vi "TagRead.vi"(7 "LabVIEW Web Service Request":refnum<class "Web Request.lvclass">, 10 "type":string, 11 "tagName":string) -> ()   [LabVIEW 2013]
doc: "TagRead returns the value of the tag specified. Specifying the type isn't required, but results in slightly faster performance."
uses:
  <vilib>/wsapi/Web Request.lvclass
  <vilib>/NI/Tag Bus/tag/Data Type.ctl
  <vilib>/NI/Tag Bus/table/data table.ctl
  <vilib>/NI/TagWebClient/API/JSON Formats/read tag value.ctl
  <vilib>/NI/TagWebClient/API/tagweb client API.lvlib
  <vilib>/NI/Tag Bus/tag/tag descriptor.lvclass
  <vilib>/NI/Tag Bus/table/data table.lvlib
  <vilib>/NI/Tag Bus/dictionary/data dictionary.lvclass
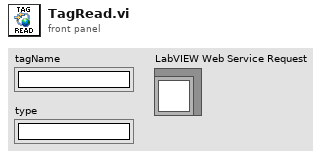
[diagram p1: front panel]
types:
  T1 = typedef "tag bus.lvlib/tag descriptor.lvclass/Data Type.ctl" = enum16{"Double", "Single", "I64", "I32", "I16", "I8", "U64", "U32", "U16", "U8", "Boolean", "String", "Array of Double", "Array of Single", "Array of I64", "Array of I32", "Array of I16", "Array of I8", "Array of U64", "Array of U32", "Array of U16", "Array of U8", "Array of Boolean", "Array of String"}
  T2 = typedef "tag bus.lvlib/data table.lvlib/data table.ctl" = cluster{"Double":dbl[], "Single":sgl[], "I64":i64[], "I32":i32[], "I16":i16[], "I8":i8[], "U64":u64[], "U32":u32[], "U16":u16[], "U8":u8[], "Boolean":bool[], "String":string[], "Array of Double":cluster{"DBL Array":dbl[]}[], "Array of Single":cluster{"SGL Array":sgl[]}[], "Array of I64":cluster{"I64 Array":i64[]}[], "Array of I32":cluster{"I32 Array":i32[]}[], "Array of I16":cluster{"I16 Array":i16[]}[], "Array of I8":cluster{"I8 Array":i8[]}[], "Array of U64":cluster{"U64 Array":u64[]}[], "Array of U32":cluster{"U32 Array":u32[]}[], "Array of U16":cluster{"U16 Array":u16[]}[], "Array of U8":cluster{"U8 Array":u8[]}[], "Array of Boolean":cluster{"Boolean Array":bool[]}[], "Array of String":cluster{"String Array":string[]}[]}
  T3 = typedef "tagweb client API.lvlib/read tag value.ctl" = cluster{"value":string}
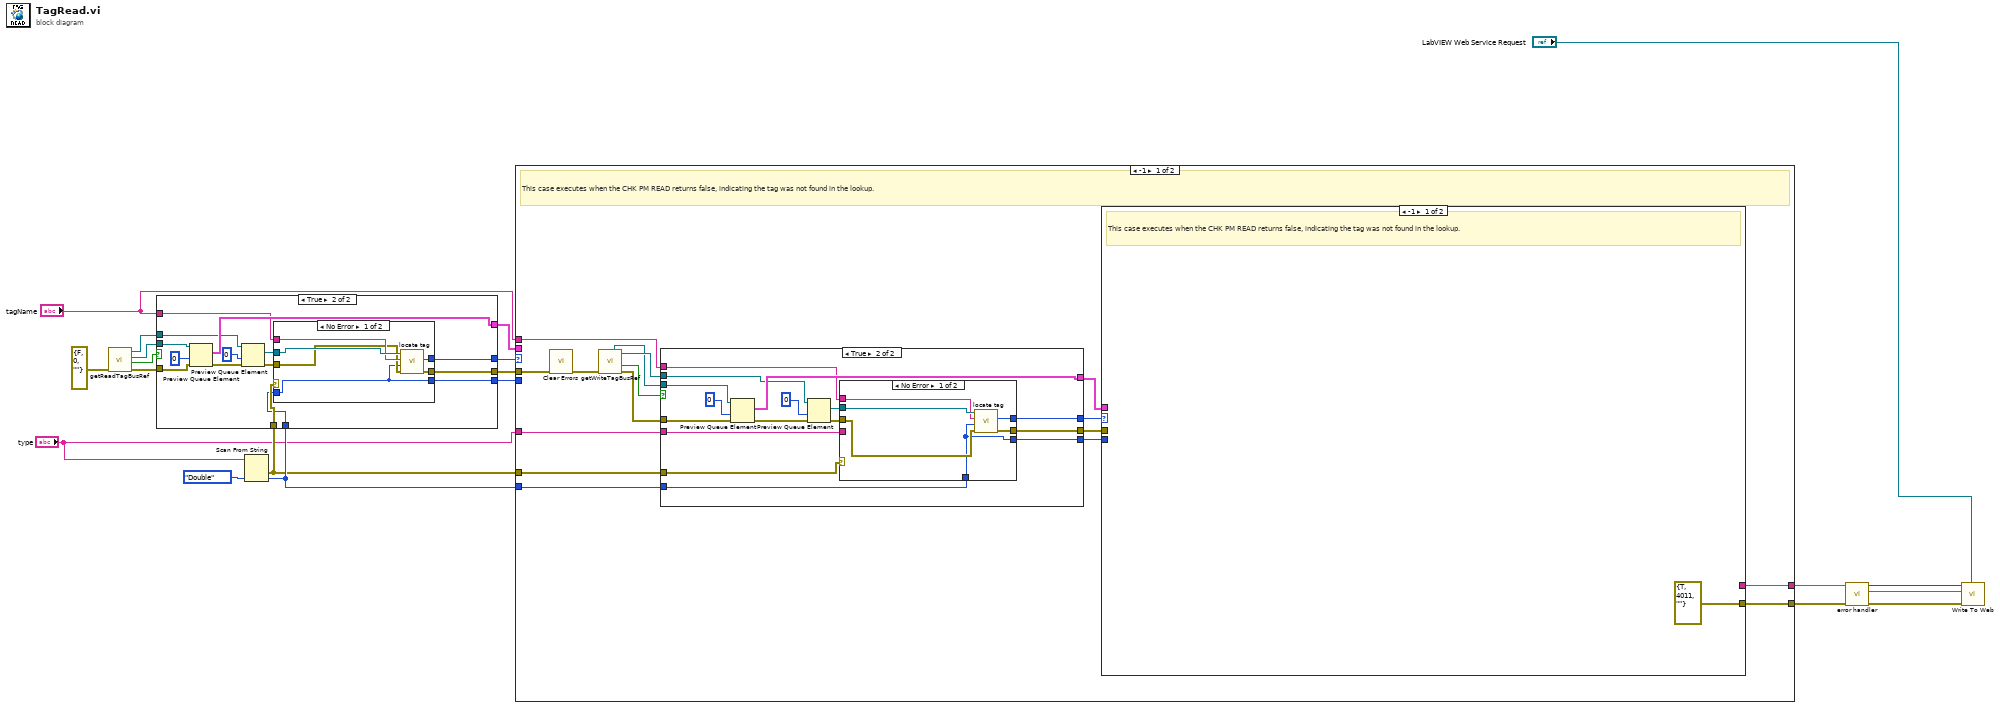
[diagram p0: block diagram]
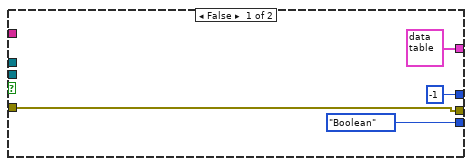
[diagram p2: hidden frame]
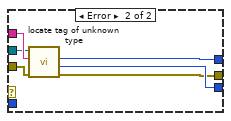
[diagram p3: hidden frame]
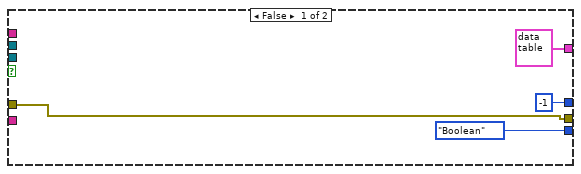
[diagram p4: hidden frame]
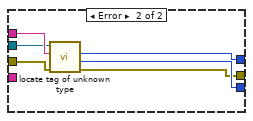
[diagram p5: hidden frame]
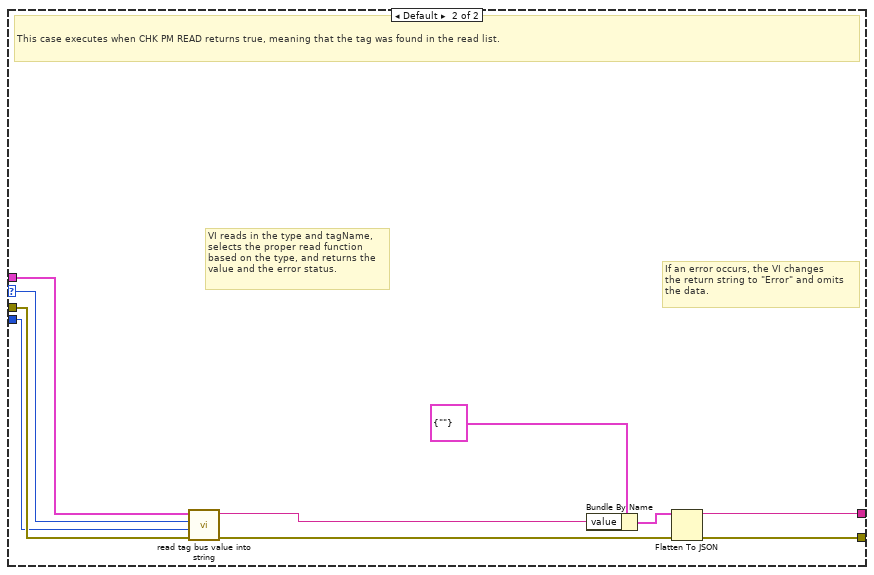
[diagram p6: hidden frame]
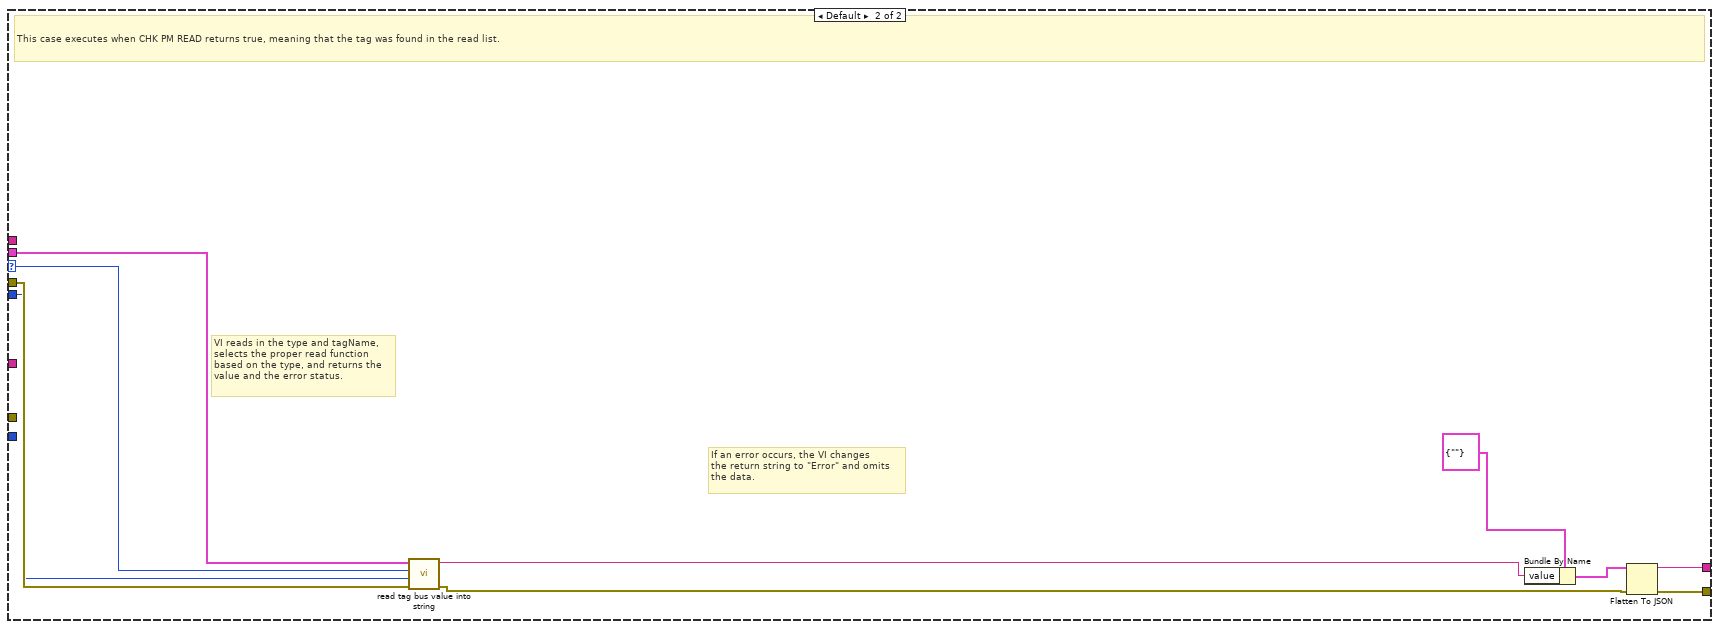
[diagram p7: hidden frame]
diagram:
  n1 = call "getReadTagBusRef.vi"("error in (no error)"=errorcluster {"status"=FALSE, "code"=0, "source"=""}) -> ("error out"=w14:errorcluster, "valid references"=w13:bool, "read data table"=w12:refnum<queue>, "read data dictionary"=w10:refnum<queue>)  [unwired: 7 in]
  n2 = Scan From String(input string="type", default 1=Data_Type."Double" ("data type")) -> (error out=w4:errorcluster, output 1=w5:T1)  [unwired: 3 in, 2 out]
  n3 = case shown="True" w13 {
    tunnel: w12 -> [_ w39]
    tunnel: [T2 {"Double"=[], "Single"=[], "I64"=[], "I32"=[], "I16"=[], "I8"=[], "U64"=[], "U32"=[], "U16"=[], "U8"=[], "Boolean"=[], "String"=[], "Array of Double"=[], "Array of Single"=[], "Array of I64"=[], "Array of I32"=[], "Array of I16"=[], "Array of I8"=[], "Array of U64"=[], "Array of U32"=[], "Array of U16"=[], "Array of U8"=[], "Array of Boolean"=[], "Array of String"=[]} ("Data Interface out") w36] -> w20
    tunnel: "tagName" -> [_ w30]
    tunnel: w14 -> [w23 w38]
    tunnel: [-1 ("index") w31] -> w19
    tunnel: [w23 w29] -> w18
    tunnel: [Data_Type."Boolean" ("data type") w32] -> w15
    tunnel: w10 -> [_ w35]
    tunnel: w4 -> [_ w26]
    tunnel: w5 -> [_ w25]
    frame False {
    }
    frame True {
      n4 = Preview Queue Element(queue=w39, timeout in ms (-1)=0, error in (no error)=w38) -> (element=w36:T2, error out=w28:errorcluster)  [unwired: 2 out]
      n5 = Preview Queue Element(queue=w35, timeout in ms (-1)=0, error in (no error)=w28) -> (element=w33:refnum<class "data dictionary.lvclass">, error out=w27:errorcluster)  [unwired: 2 out]
      n6 = case shown="No Error" w26 {
        tunnel: w33 -> [w45 w50]
        tunnel: [w40 w48] -> w32
        tunnel: [w44 w49] -> w31
        tunnel: w30 -> [w43 w51]
        tunnel: [w42 w46] -> w29
        tunnel: w27 -> [w41 w47]
        tunnel: w25 -> [w40 _]
        frame No Error {
          n7 = call <vilib>:"locate tag.vi"("error in"=w41, "data type"=w40, "name"=w43, "data dictionary in"=w45) -> ("error out"=w42:errorcluster, "index"=w44:i32)  [unwired: 5 in, 1 out]
        }
        frame Error {
          n8 = call <vilib>:"locate tag of unknown type.vi"("error in"=w47, "name"=w51, "data dictionary in"=w50) -> ("error out"=w46:errorcluster, "data type"=w48:T1, "index"=w49:i32)  [unwired: 5 in, 1 out]
        }
      }
    }
  }
  n9 = case shown="-1" w19 {
    selector: w19 -> [_ w112]
    tunnel: "tagName" -> [w64 _]
    tunnel: w18 -> [w57 w119]
    tunnel: [w58 w115] -> w17
    tunnel: [w55 w117] -> w16
    tunnel: w20 -> [_ w114]
    tunnel: w15 -> [_ w113]
    tunnel: "type" -> [w63 _]
    tunnel: w5 -> [w53 _]
    tunnel: w4 -> [w52 _]
    frame -1 {
      # "This case executes when the CHK PM READ returns false, indicating the tag was not found in the lookup."
      n10 = call <vilib>:"Clear Errors.vi"("error in (no error)"=w57) -> ("error out"=w56:errorcluster)  [unwired: 6 in]
      n11 = call "getWriteTagBusRef.vi"("error in"=w56) -> ("error out"=w65:errorcluster, "valid references"=w66:bool, "write data dictionary"=w67:refnum<queue>, "actual write data table"=w54:refnum<queue>)  [unwired: 6 in, 1 out]
      n12 = case shown="True" w66 {
        tunnel: w54 -> [_ w87]
        tunnel: [T2 {"Double"=[], "Single"=[], "I64"=[], "I32"=[], "I16"=[], "I8"=[], "U64"=[], "U32"=[], "U16"=[], "U8"=[], "Boolean"=[], "String"=[], "Array of Double"=[], "Array of Single"=[], "Array of I64"=[], "Array of I32"=[], "Array of I16"=[], "Array of I8"=[], "Array of U64"=[], "Array of U32"=[], "Array of U16"=[], "Array of U8"=[], "Array of Boolean"=[], "Array of String"=[]} ("Data Interface out") w84] -> w61
        tunnel: w64 -> [_ w77]
        tunnel: w65 -> [w70 w86]
        tunnel: [-1 ("index") w78] -> w60
        tunnel: [w70 w76] -> w59
        tunnel: [Data_Type."Boolean" ("data type") w79] -> w62
        tunnel: w67 -> [_ w83]
        tunnel: w63 -> [_ w81]
        tunnel: w53 -> [_ w73]
        tunnel: w52 -> [_ w72]
        frame False {
        }
        frame True {
          n13 = Preview Queue Element(queue=w87, timeout in ms (-1)=0, error in (no error)=w86) -> (element=w84:T2, error out=w75:errorcluster)  [unwired: 2 out]
          n14 = Preview Queue Element(queue=w83, timeout in ms (-1)=0, error in (no error)=w75) -> (element=w80:refnum<class "data dictionary.lvclass">, error out=w74:errorcluster)  [unwired: 2 out]
          n15 = case shown="No Error" w72 {
            tunnel: w81 -> [_ _]
            tunnel: w80 -> [w93 w98]
            tunnel: [w88 w96] -> w79
            tunnel: [w92 w97] -> w78
            tunnel: w77 -> [w91 w99]
            tunnel: [w90 w94] -> w76
            tunnel: w74 -> [w89 w95]
            tunnel: w73 -> [w88 _]
            frame No Error {
              n16 = call <vilib>:"locate tag.vi"("error in"=w89, "data type"=w88, "name"=w91, "data dictionary in"=w93) -> ("error out"=w90:errorcluster, "index"=w92:i32)  [unwired: 5 in, 1 out]
            }
            frame Error {
              n17 = call <vilib>:"locate tag of unknown type.vi"("error in"=w95, "name"=w99, "data dictionary in"=w98) -> ("error out"=w94:errorcluster, "data type"=w96:T1, "index"=w97:i32)  [unwired: 5 in, 1 out]
            }
          }
        }
      }
      n18 = case shown="-1" w60 {
        selector: w60 -> [_ w102]
        tunnel: w59 -> [_ w107]
        tunnel: [errorcluster {"status"=TRUE, "code"=4011, "source"=""} ("error in (no error)") w108] -> w58
        tunnel: [_ w109] -> w55
        tunnel: w61 -> [_ w104]
        tunnel: w62 -> [_ w103]
        frame -1 {
          # "This case executes when the CHK PM READ returns false, indicating the tag was not found in the lookup."
        }
        frame Default {
          # "If an error occurs, the VI changes\nthe return string to \"Error\" and omits\nthe data."
          # "VI reads in the type and tagName,\nselects the proper read function\nbased on the type, and returns the\nvalue and the error status."
          # "This case executes when CHK PM READ returns true, meaning that the tag was found in the read list."
          n19 = call "read tag bus value into string.vi"("error in (no error)"=w107, "data type"=w103, "index"=w102, "data table"=w104) -> ("error out"=w106:errorcluster, "Value"=w105:string)  [unwired: 6 in]
          n20 = Bundle By Name(cluster=T3 {"value"=""} ("tag value"), "value"=w105) -> (w110:T3)
          n21 = Flatten To JSON(anything=w110, error in (no error)=w106) -> (JSON string=w109:string, 11:w108:errorcluster)  [unwired: 1 in]
        }
      }
    }
    frame Default {
      # "If an error occurs, the VI changes\nthe return string to \"Error\" and omits\nthe data."
      # "VI reads in the type and tagName,\nselects the proper read function\nbased on the type, and returns the\nvalue and the error status."
      # "This case executes when CHK PM READ returns true, meaning that the tag was found in the read list."
      n22 = call "read tag bus value into string.vi"("error in (no error)"=w119, "data type"=w113, "index"=w112, "data table"=w114) -> ("error out"=w116:errorcluster, "Value"=w120:string)  [unwired: 6 in]
      n23 = Bundle By Name(cluster=T3 {"value"=""} ("tag value"), "value"=w120) -> (w118:T3)
      n24 = Flatten To JSON(anything=w118, error in (no error)=w116) -> (JSON string=w117:string, 11:w115:errorcluster)  [unwired: 1 in]
    }
  }
  n25 = call "error handler.vi"("error in (no error)"=w17, "Success Message"=w16) -> ("error out"=w9:errorcluster, "Response String"=w7:string, "Response Code"=w8:i32)  [unwired: 7 in]
  n26 = call <vilib>:"Write To Web.vi"("Web Request in"="LabVIEW Web Service Request", "error in"=w9, "Response String"=w7, "Response Code"=w8) -> ()  [unwired: 8 in]
